vi "Read Display Settings from File.vi"(8 "error in (no error)":errorcluster, 11 "State in":T4 caption="State" {"Centroid"."Y Centroid" format="%.2f"; "Centroid"."X Centroid" format="%.2f"; "ROI"."Contours"."Type" items=["No Selection", "Point", "Line", "Rectangle", "Oval", "Polygon", "Freehand Region", "Annulus", "Unused2", "Unused3", "Broken Line", "Freehand Line", "Rotated Rectangle"]}) -> (0 "error out":errorcluster, 3 "State out":T4 caption="State" {"Centroid"."Y Centroid" format="%.2f"; "Centroid"."X Centroid" format="%.2f"; "ROI"."Contours"."Type" items=["No Selection", "Point", "Line", "Rectangle", "Oval", "Polygon", "Freehand Region", "Annulus", "Unused2", "Unused3", "Broken Line", "Freehand Line", "Rotated Rectangle"]})   [LabVIEW 2009, in "POLARIS IMAQ Display.xctl"]
doc: "Retreat saved parameters of POLARIS IMAQ Display and fill XControl state cluster . \n[in | out ] State cluster of XControl\nVI fills dummy controls ROI, SavedROI, Display with values from file and maps they in XControl State cluster.\nThe dummy contorl must have the same names like dummy controls in Write Display Settings 2 File.vi\n\n\nauthor: Alexander Kessler, Helmholtz-Institut-Jena \nmaintainer: Alexander Kessler: alexander.kessler@uni-jena.de\n\n\n\nLicense Agreement for this software:\n\nCopyright (C)\nHelmholtz-Institut-Jena\nFröbelstieg 3\n07743 Jena\nGermany\n\nThis program is free software; you can redistribute it and/or modify it under the terms of the GNU General Public License as published by the Free Software Foundation; either version 2 of the license, or (at your option) any later version.\n\nThis program is distributed in the hope that it will be useful, but WITHOUT ANY WARRANTY; without even the implied warranty of MERCHANTABILITY or FITNESS FOR A PARTICULAR PURPOSE. See the GNU General License for more details (http://www.gnu.org)."
uses:
  POLARIS IMAQ Display.xctl
  Named ROI.ctl
  State.ctl
  IMAQdx Cam/IMAQdx Cam.lvclass
  Properties/ImageSource.ctl
  <vilib>/vision/Image Controls.llb/IMAQ Image.ctl
  DisplaySettings.ctl
  Analyze Classes/Analyze BaseClass/Analyze BaseClass.lvclass
  Palette.ctl
  Utility/POLARIS Vision utility.lvlib
panel:
  in  "Pallete":T1={"Teiler"=1, "Palette Type"=0} {"Teiler" min=1 max=5; "Palette Type" items=["Grayscale", "Binary", "Gradient", "Rainbow", "Temperature", "User Defined"]}
  in  "Image Center":cluster{"X":u32, "Y":u32}
  in  "Zoom":cluster{"X":i32, "Y":i32}
  in  "ROI":T2 {"Contours"."Type" items=["No Selection", "Point", "Line", "Rectangle", "Oval", "Polygon", "Freehand Region", "Annulus", "Unused2", "Unused3", "Broken Line", "Freehand Line", "Rotated Rectangle"]}
  in  "Display settings":T3={"Min. Thresh."=0.0, "X"=0.0, "Y"=0.0, "ShowLineout"=FALSE, "ScaleParts"=10, "ShowLegende"=FALSE, "Target Cross"=FALSE, "Centroid Cross"=FALSE, "Target color"=16777226, "Centroid color"=16711680, "calibr. mm/px"=0.0}
  in  "Saved ROIs":T7[](array[typedef])
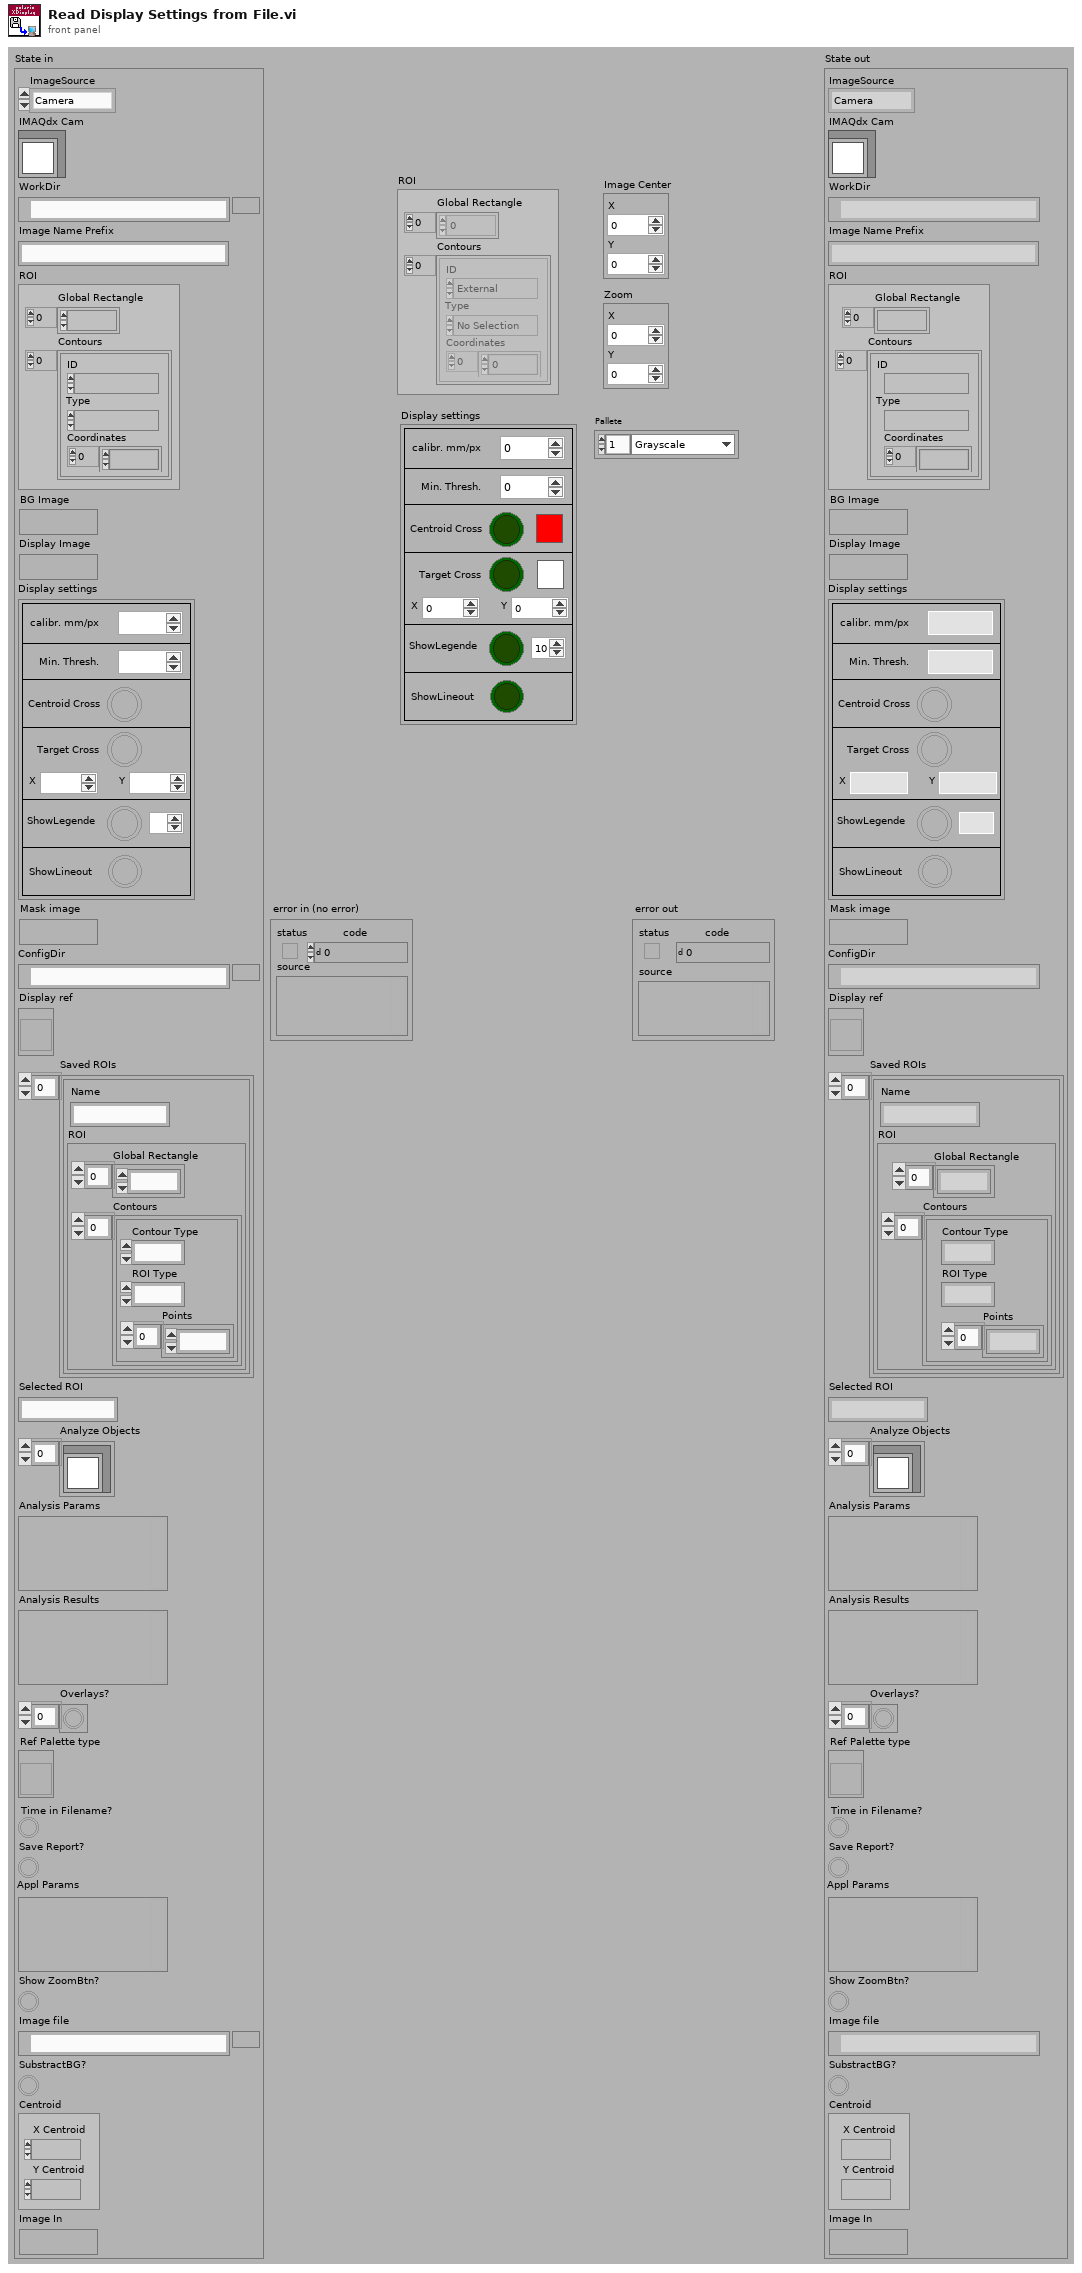
[diagram p1: front panel]
types:
  T1 = typedef "POLARIS IMAQ Display.xctl/Palette.ctl" = cluster{"Teiler":i32, "Palette Type":u32}
  T2 = typedef "ROI Descriptor" = cluster{"Global Rectangle":i32[], "Contours":cluster{"ID":enum32{"External", "Internal"}, "Type":u32, "Coordinates":i32[]}[]}
  T3 = typedef "POLARIS IMAQ Display.xctl/DisplaySettings.ctl" = cluster{"Min. Thresh.":sgl, "X":dbl, "Y":dbl, "ShowLineout":bool, "ScaleParts":i32, "ShowLegende":bool, "Target Cross":bool, "Centroid Cross":bool, "Target color":u32, "Centroid color":u32, "calibr. mm/px":sgl}
  T4 = typedef "POLARIS IMAQ Display.xctl/State.ctl" = cluster{"ImageSource":T5, "IMAQdx Cam":refnum<class "IMAQdx Cam.lvclass">, "WorkDir":path, "Image Name Prefix":string, "ROI":T2, "BG Image":T6, "Display Image":T6, "Display settings":T3, "Mask image":T6, "ConfigDir":path, "Display ref":refnum<vi>, "Saved ROIs":T7[], "Selected ROI":string, "Analyze Objects":refnum<class "Analyze BaseClass.lvclass">[], "Analysis Params":variant, "Analysis Results":variant, "Overlays?":bool[], "Ref Palette type":refnum<vi>, "Time in Filename?":bool, "Save Report?":bool, "Appl Params":variant, "Show ZoomBtn?":bool, "Image file":path, "SubstractBG?":bool, "Centroid":cluster{"X Centroid":sgl, "Y Centroid":sgl}, "Image In":T6}
  T5 = typedef "POLARIS IMAQ Display.xctl/ImageSource.ctl" = enum16{"Camera", "File"}
  T6 = typedef "IMAQ Image.ctl" = refnum<image>
  T7 = typedef "POLARIS IMAQ Display.xctl/Named ROI.ctl" = cluster{"ROI":cluster{"Global Rectangle":i32[], "Contours":cluster{"Contour Type":u32, "ROI Type":u32, "Points":i32[]}[]}, "Name":string}
  T8 = typedef "IMAQdx.ctl" = refnum<k21>
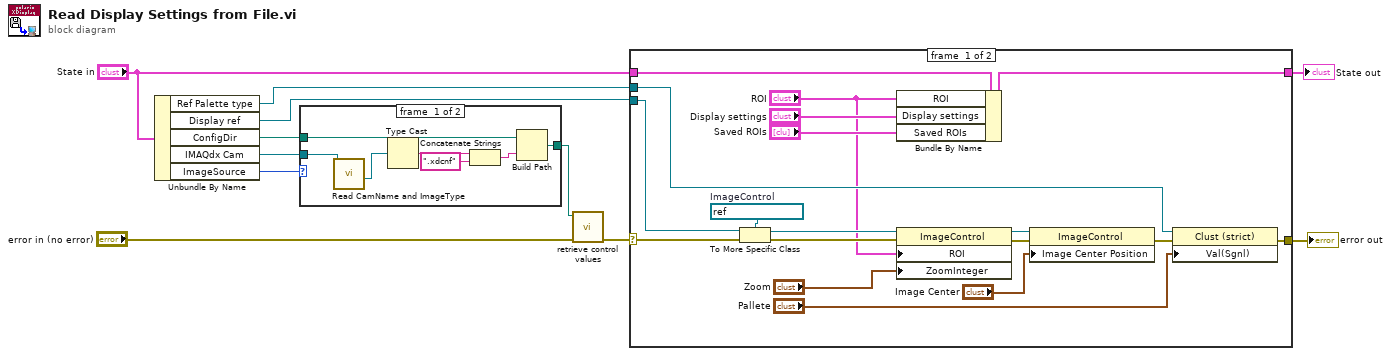
[diagram p0: block diagram]
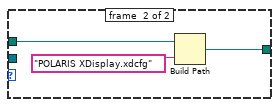
[diagram p2: hidden frame]
diagram:
  n1 = Unbundle By Name("State in") -> ("Ref Palette type"=w1:refnum<vi>, "Display ref"=w2:refnum<vi>, "ConfigDir"=w6:path, "IMAQdx Cam"=w7:refnum<class "IMAQdx Cam.lvclass">, "ImageSource"=w3:T5)
  n2 = case shown="\"File\"" w3 {
    tunnel: w7 -> [w18 _]
    tunnel: w6 -> [w17 w20]
    tunnel: [w12 w19] -> w4
    frame #0 {
      n3 = call-dynamic "Read CamName and ImageType.vi"("IMAQdx Cam in"=w18) -> ("Camera"=w13:T8)  [unwired: 7 in, 3 out]
      n4 = Type Cast(x=w13) -> (*(type *) &x=w16:string)  [unwired: 1 in]
      n5 = Concatenate Strings(w16, ".xdcnf" ("string")) -> (w15:string)
      n6 = Build Path(base path=w17, name or relative path=w15) -> (appended path=w12:path)
    }
    frame #1 {
      n7 = Build Path(base path=w20, name or relative path="POLARIS XDisplay.xdcfg") -> (appended path=w19:path)
    }
  }
  n8 = call "retrieve control values.vi"("error in (no error)"="error in (no error)", "path"=w4) -> ("error out"=w10:errorcluster)  [unwired: 8 in, 1 out]
  n9 = case shown="No Error" w10 {
    selector: w10 -> [w33 w41]
    tunnel: [w30 w41] -> w9
    tunnel: [w39 w40] -> w8
    tunnel: "State in" -> [w38 w40]
    tunnel: w2 -> [w31 _]
    tunnel: w1 -> [w29 _]
    frame #0 {
      w26 = refnum<vi> refnum  # ImageControl
      n10 = To More Specific Class(target class=w26, reference=w31, error in=w33) -> (specific class reference=w34:refnum<vi>, error out=w35:errorcluster)
      n11 = Bundle By Name(cluster=w38, "ROI"="ROI", "Display settings"="Display settings", "Saved ROIs"="Saved ROIs") -> (w39:T4)
      n12 = property class="ImageControl"(reference=w34, error in=w35, "ROI"="ROI", "ZoomInteger"="Zoom") -> (reference out=w22:refnum<vi>, error out=w24:errorcluster)
      n13 = property class="ImageControl"(reference=w22, error in=w24, "Image Center Position"="Image Center") -> (error out=w23:errorcluster)  [unwired: 1 out]
      n14 = property class="Clust (strict)"(reference=w29, error in=w23, "Val(Sgnl)"="Pallete") -> (error out=w30:errorcluster)  [unwired: 1 out]
    }
    frame #1 {
    }
  }
  "error out" <- w9
  "State out" <- w8
